vi "SaveFileOnProcessor.vi"(11 "Save":cluster{"fileName":string, "Code":string}) -> (3 "Code":string)   [LabVIEW 2020]
panel:
  # "import os\n\nfile = open('Main.py','wb')\ntext = file.write(b'\\x66\\x6F\\x72\\x20\\x69\\x20\\x69\\x6E\\x20\\x72\\x61\\x6E\\x67\\x65\\x28\\x31\\x30\\x29\\x3A\\x0A\\x20\\x20\\x20\\x20\\x20\\x70\\x72\\x69\\x6E\\x74\\x28\\x69\\x29\\x0A')\nfile.close()\ntext"
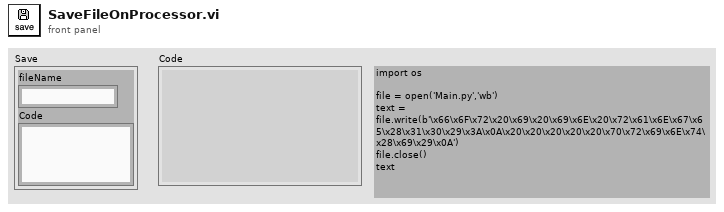
[diagram p1: front panel]
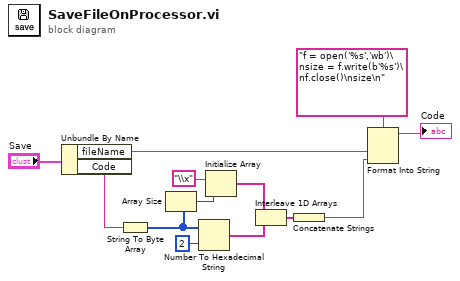
[diagram p0: block diagram]
diagram:
  n1 = Unbundle By Name("Save") -> ("fileName"=w11:string, "Code"=w9:string)
  n2 = String To Byte Array(string=w9) -> (unsigned byte array=w6:u8[])
  n3 = Array Size(array=w6) -> (size(s)=w5:i32)
  n4 = Number To Hexadecimal String(1:i16 2 ("width (-)"), 2:w6) -> (0:w3:string[])
  n5 = Initialize Array("\\x", w5) -> (w4:string[])
  n6 = Interleave 1D Arrays(w4, w3) -> (w2:string[])
  n7 = Concatenate Strings(w2) -> (w1:string)
  n8 = Format Into String(format string="f = open('%s','wb')\nsize = f.write(b'%s')\nf.close()\nsize\n", w11, w1) -> (resulting string=→"Code":string)  [unwired: 2 in, 1 out]
